vi "getDriveEncoders.vi"() -> (0 "Rate FPS":cluster{"Left":dbl, "Right":dbl}, 1 "Rate IPS":cluster{"Left":dbl, "Right":dbl}, 2 "Average FPS":dbl, 3 "Distance":cluster{"Left":dbl, "Right":dbl})   [LabVIEW 2012]
panel:
  in  "Encoder Bias":cluster{"Distance":dbl, "Distance":dbl}={"Distance"=0.99, "Distance"=1.0}
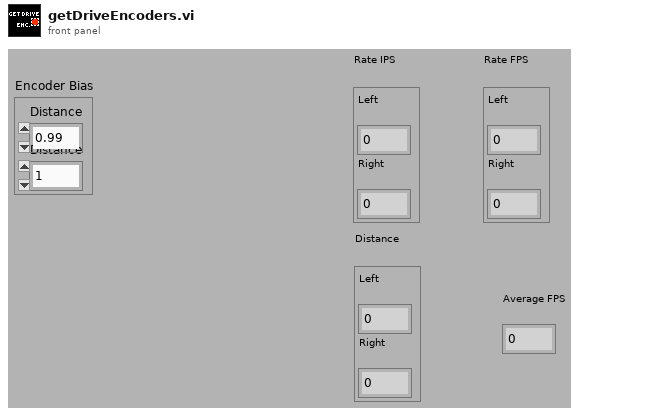
[diagram p1: front panel]
types:
  T1 = typedef "WPI_EncoderDevRef.ctl" = cluster{"DevStatus":errorcluster, "EncoderIndex":T2, "CounterIndex":T3, "DistancePerCount":dbl, "Decoding Type":T4}
  T2 = typedef "FPGA_EncoderIdx.ctl" = enum8{"Enc 0", "Enc 1", "Enc 2", "Enc 3", "Invalid"}
  T3 = typedef "FPGA_CounterCtrSystemIndex.ctl" = enum8{"Ctr 0", "Ctr 1", "Ctr 2", "Ctr 3", "Ctr 4", "Ctr 5", "Ctr 6", "Ctr 7", "Invalid"}
  T4 = typedef "WPI_EncoderType.ctl" = enum16{"1x", "2x", "4x"}
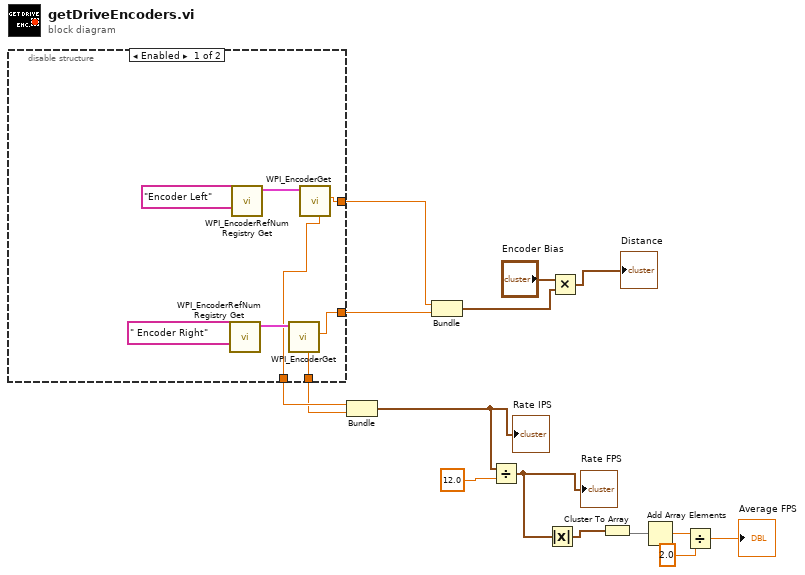
[diagram p0: block diagram]
diagram:
  n1 = disable-structure shown="Enabled" {
    disable-tunnel: [w18 _] -> w8
    disable-tunnel: [w23 _] -> w7
    disable-tunnel: [w19 _] -> w5
    disable-tunnel: [w22 _] -> w4
    frame Enabled {
      n2 = call <vilib>:"WPI_EncoderRefNum Registry Get.vi"("refnum name"=" Encoder Right") -> ("EncoderDevRef"=w21:T1)  [unwired: 1 in, 9 out]
      n3 = call <vilib>:"WPI_EncoderRefNum Registry Get.vi"("refnum name"="Encoder Left") -> ("EncoderDevRef"=w20:T1)  [unwired: 1 in, 9 out]
      n4 = call <vilib>:"WPI_EncoderGet.vi"("EncoderDevRef"=w21) -> ("Distance"=w23:dbl, "Rate"=w22:dbl)  [unwired: 1 in, 8 out]
      n5 = call <vilib>:"WPI_EncoderGet.vi"("EncoderDevRef"=w20) -> ("Distance"=w18:dbl, "Rate"=w19:dbl)  [unwired: 1 in, 8 out]
    }
    frame Disabled {
    }
  }
  n6 = Bundle("Rate"=w5, "Rate"=w4) -> (w6:cluster{"Rate":dbl, "Rate":dbl})  [unwired: 1 out]
  "Rate IPS" <- w6
  n7 = Bundle("Distance"=w8, "Distance"=w7) -> (w2:cluster{"Distance":dbl, "Distance":dbl})  [unwired: 1 out]
  n8 = Divide(x=w6, y=12.0) -> (x/y=w9:cluster{"Rate":dbl, "Rate":dbl})
  "Rate FPS" <- w9
  n9 = Absolute Value(x=w9) -> (abs(x)=w10:cluster{"Rate":dbl, "Rate":dbl})
  n10 = Multiply(x="Encoder Bias", y=w2) -> (x*y=→"Distance":cluster{"Distance":dbl, "Distance":dbl})
  n11 = Cluster To Array(cluster=w10) -> (array=w14:dbl[])
  n12 = Add Array Elements(numeric array=w14) -> (sum=w13:dbl)
  n13 = Divide(x=w13, y=2.0) -> (x/y=→"Average FPS":dbl)
